vi "Increment Limiter.vi"(8 "Increment":dbl, 11 "Ref":dbl) -> (3 "Output":dbl)   [LabVIEW 2010]
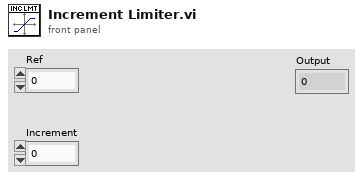
[diagram p1: front panel]
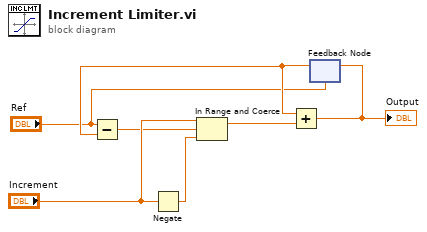
[diagram p0: block diagram]
diagram:
  n1 = Negate(x="Increment") -> (-x=w6:dbl)
  n2 = feedback #1("Ref") -> (w3:dbl)
  n3 = Subtract(x="Ref", y=w3) -> (x-y=w2:dbl)
  n4 = In Range and Coerce(upper limit="Increment", x=w2, lower limit=w6) -> (coerced(x)=w5:dbl)  [unwired: 1 out]
  n5 = Add(x=w3, y=w5) -> (x+y=w4:dbl)
  "Output" <- w4
  n6 = feedback-in #1(w4) -> ()
